vi "Reserve Drive.vi"(7 "Description":string="Reserve", 8 "Command Info":T1, 10 "Command Name":string) -> (0 "Command Info":T1)   [LabVIEW 2019]
doc: "Reserve the Drive subsystem. This is used when multiple subsystems are needed for a Macro and you want exclusive control for the duration."
uses:
  <vilib>/Rock Robotics/WPI/Framework/Command Status Info.ctl
  <vilib>/Rock Robotics/WPI/Framework/Completion Status.ctl
  <vilib>/Rock Robotics/WPI/Framework/Completion Notifier.ctl
  Implementation/Drive Setpoints.ctl
  Implementation/Drive Operations.ctl
  Support Code/Single Cmd Info.ctl
  <vilib>/picture/picture.llb/imagedata.ctl
  Support Code/types/Limits.ctl
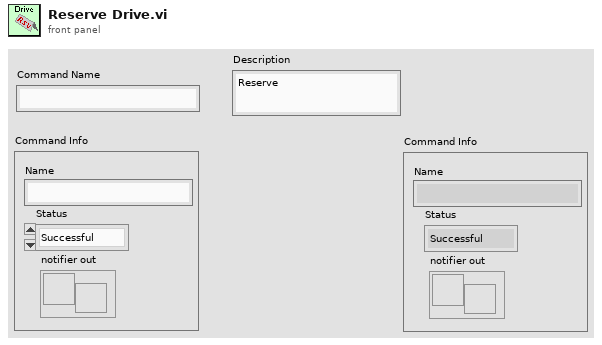
[diagram p1: front panel]
types:
  T1 = typedef "Command Status Info.ctl" = cluster{"Name":string, "Status":T2, "notifier out":T3}
  T2 = typedef "Completion Status.ctl" = enum16{"Successful", "Aborted", "Incomplete"}
  T3 = typedef "Completion Notifier.ctl" = refnum<notifier>
  T4 = typedef "Drive Setpoints.ctl" = cluster{"Operation":T5, "Setpoints":cluster{"Left Setpoint":dbl, "Right Setpoint":dbl}, "Path stuff":cluster{"Direction":cluster{"Reverse Path":bool, "Robot Backwards":bool}, "Traj Vel Points":cluster{"V":dbl, "th":dbl}[], "Commands":cluster{"Time (s)":dbl, T6, bool}[], "Limits":cluster{"Sample Period (s)":dbl, "Limits":T8, "Conditions":cluster{"vInitial (fps)":dbl, "vFinal (fps)":dbl}, cluster{dbl[], bool[]}}}}
  T5 = typedef "Drive Operations.ctl" = enum16{"Reserve", "Read Current", "Immediate", "Play Path"}
  T6 = typedef "Single Cmd Info.ctl" = cluster{"Name":string, "CPTM.DataType":variant, "All Control Values Variant":cluster{"Name":string, "Variant Data":variant}[], "icon full":T7, "icon scaled":T7, "Path":path, "Subsystem Color":u32}
  T7 = typedef "imagedata.ctl" = cluster{"image type":i32, "image depth":i32, "image":u8[], "mask":u8[], "colors":u32[], "Rectangle":cluster{"left":i16, "top":i16, "right":i16, "bottom":i16}}
  T8 = typedef "Limits.ctl" = cluster{"Velocity (fps)":dbl, "Accel (fps^2)":dbl, "Jerk (fps^3)":dbl, "StoopidFast (fps)":dbl}
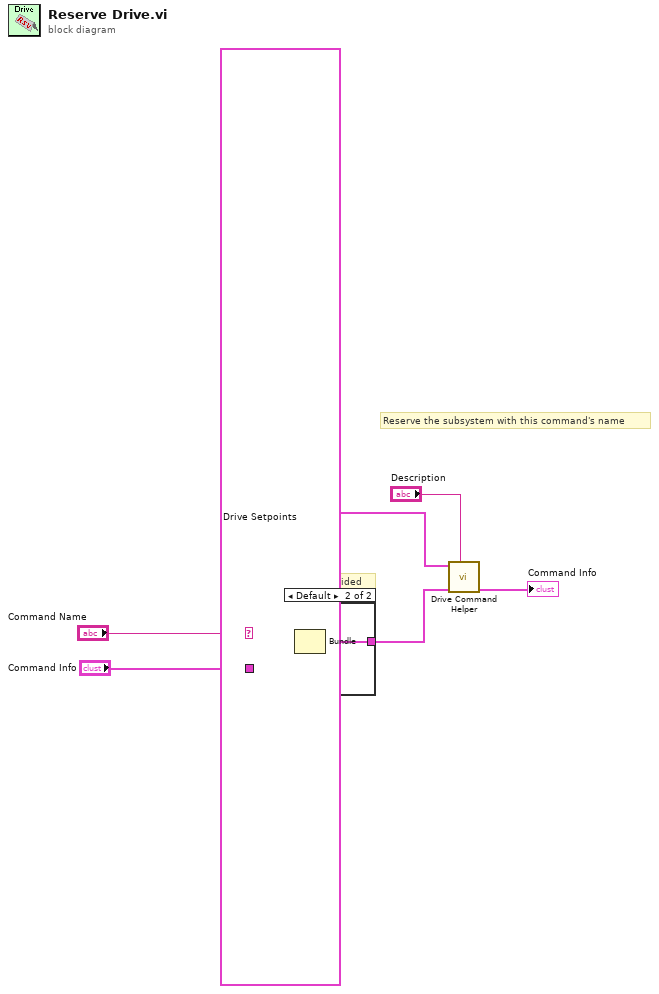
[diagram p0: block diagram]
diagram:
  # "Update name, if provided"
  # "Reserve the subsystem with this command's name"
  n1 = case shown="Default" "Command Name" {
    selector: "Command Name" -> [_ w8]
    tunnel: "Command Info" -> [w7 w10]
    tunnel: [w7 w9] -> w3
    frame "" {
    }
    frame Default {
      n2 = Bundle(cluster=w10, "Name"=w8) -> (w9:T1)  [unwired: 2 in]
    }
  }
  n3 = call "Drive Command Helper.vi"("Description"="Description", "Command Info In"=w3, "SubSystem Data"=T4 {"Operation"=enum."Reserve", "Setpoints"={"Left Setpoint"=0.0, "Right Setpoint"=0.0}, "Path stuff"={"Direction"={"Reverse Path"=FALSE, "Robot Backwards"=FALSE}, "Traj Vel Points"=[], "Commands"=[], "Limits"={"Sample Period (s)"=0.0, "Limits"={"Velocity (fps)"=0.0, "Accel (fps^2)"=0.0, "Jerk (fps^3)"=0.0, "StoopidFast (fps)"=0.0}, "Conditions"={"vInitial (fps)"=0.0, "vFinal (fps)"=0.0}, {[], []}}}}) -> ("Command Info Out"=→"Command Info":T1)  [unwired: 6 in, 2 out]
